vi "Periodic Extend.vi"(8 "error in (no error)":errorcluster, 9 "Waveform in":waveform(dbl)) -> (0 "error out":errorcluster, 1 "Waveform out":waveform(dbl), 2 "No. of points":i32)   [LabVIEW 2019]
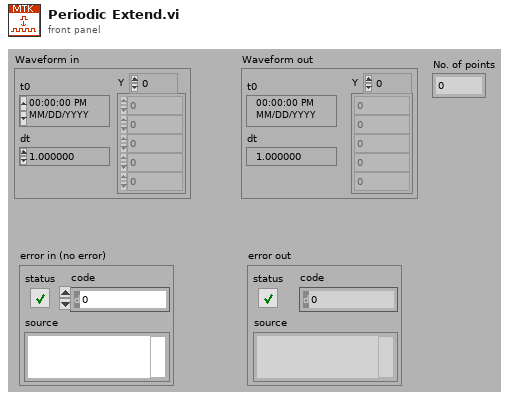
[diagram p1: front panel]
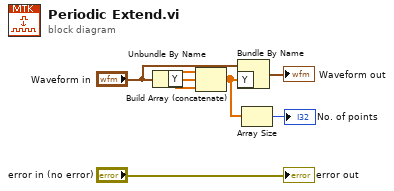
[diagram p0: block diagram]
diagram:
  n1 = Unbundle By Name("Waveform in") -> ("Y"=w4:dbl[])
  n2 = Build Array (concatenate)(w4, w4, w4) -> (w2:dbl[])
  n3 = Bundle By Name(cluster="Waveform in", "Y"=w2) -> (→"Waveform out":waveform(dbl))
  n4 = Array Size(array=w2) -> (size(s)=→"No. of points":i32)
  "error out" <- "error in (no error)"
